vi "Flatten.vi"(6 "Indent":i32, 7 "Linked List in":refnum<class "Linked List.lvclass">, 8 "error in (no error)":errorcluster, 9 "Child IDs":string[](array[string]), 11 "IPersist in":refnum<class "IPersist.lvclass">) -> (0 "error out":errorcluster, 1 "Flattened Linked List":string[](array[string]), 3 "IPersist out":refnum<class "IPersist.lvclass">, 5 "Linked List out":refnum<class "Linked List.lvclass">)   [LabVIEW 2017, in "Linked Lists.lvlib" / "Linked List.lvclass"]
uses:
  <vilib>/gpm_packages/@cs/linked-list/Source/Linked List/Linked List/Linked List.lvclass
  <vilib>/gpm_packages/@cs/persistence/source/IPersist/IPersist.lvclass
  <vilib>/gpm_packages/@cs/linked-list/Source/String Manipulation/String Manipulation.lvlib
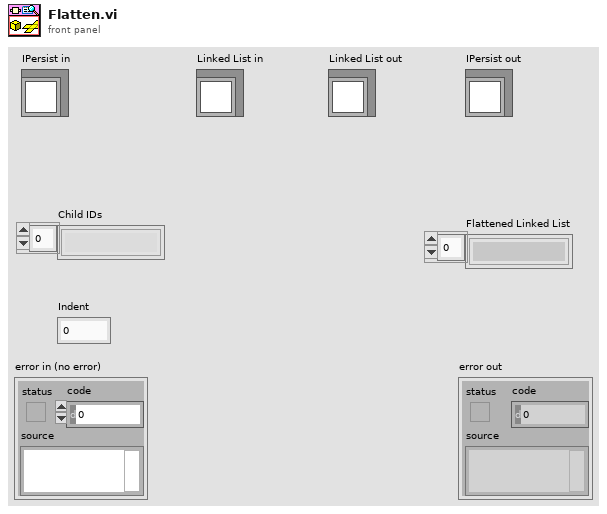
[diagram p1: front panel]
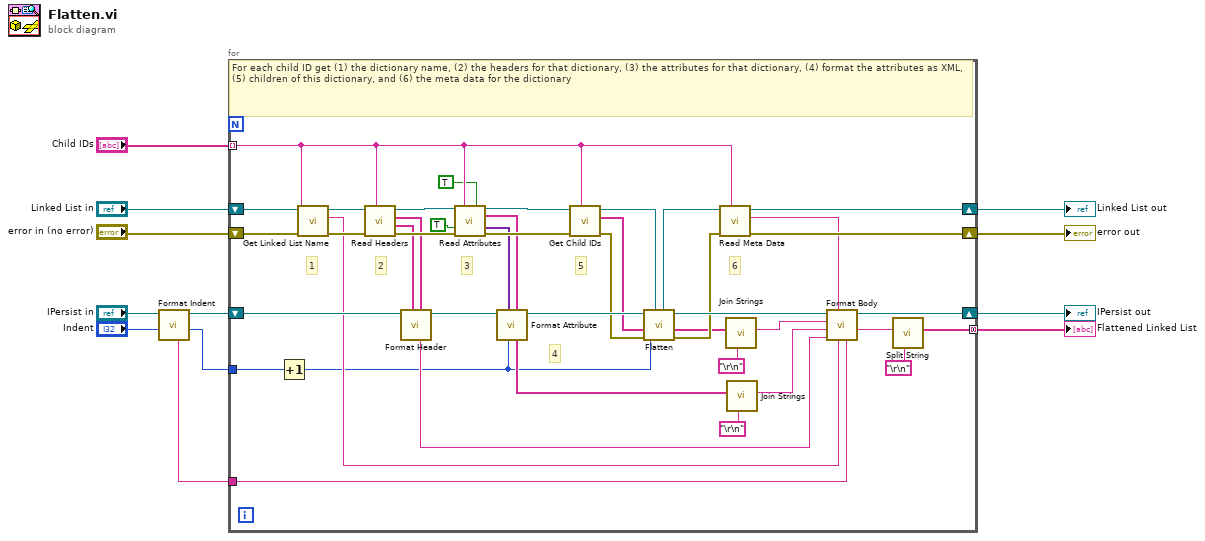
[diagram p0: block diagram]
diagram:
  n1 = call-dynamic "Format Indent.vi"("Indent"="Indent", "IPersist in"="IPersist in") -> ("Indent out"=w11:i32, "IPersist out"=w12:refnum<class "IPersist.lvclass">, "Indent XML"=w10:string)  [unwired: 7 in]
  n2 = for {
    shift-right: [w47] -> w1
    shift-left: "Linked List in" -> [w50]
    shift-right: [w36] -> w3
    shift-left: w12 -> [w45]
    shift-right: [w41] -> w2
    shift-left: "error in (no error)" -> [w49]
    tunnel: w11 -> [w37]
    tunnel: w10 -> [w27]
    tunnel: "Child IDs" -> [w46] mode=indexing
    tunnel: [w25] -> w4 mode=concatenating
    # "4"
    # "6"
    # "5"
    # "3"
    # "2"
    # "1"
    # "For each child ID get (1) the dictionary name, (2) the headers for that dictionary, (3) the attributes for that dictionary, (4) format the attributes as XML, (5) children of this dictionary, and (6) the meta data for the dictionary"
    n3 = Increment(x=w37) -> (x+1=w13:i32)
    n4 = call-dynamic "Get Linked List Name.vi"("error in (no error)"=w49, "Unique ID"=w46, "Linked List in"=w50) -> ("error out"=w53:errorcluster, "Linked List Name"=w28:string, "Linked List out"=w54:refnum<class "Linked List.lvclass">)  [unwired: 5 in, 1 out]
    n5 = call-dynamic "Read Headers.vi"("Linked List ID"=w46, "error in (no error)"=w53, "Linked List in"=w54) -> ("error out"=w51:errorcluster, "Header Values"=w44:string[], "Header Names"=w43:string[], "Linked List out"=w52:refnum<class "Linked List.lvclass">)  [unwired: 4 in, 1 out]
    n6 = call-dynamic "Format Header.vi"("Name"=w43, "Value"=w44, "IPersist in"=w45) -> ("IPersist out"=w40:refnum<class "IPersist.lvclass">, "Header"=w29:string)  [unwired: 7 in]
    n7 = call-dynamic "Read Attributes.vi"("Linked List in"=w52, "Linked List ID"=w46, "Include Private?"=TRUE, "Flatten Pointer?"=TRUE, "error in (no error)"=w51) -> ("Linked List out"=w48:refnum<class "Linked List.lvclass">, "Attribute Names out"=w38:string[], "Attributes"=w39:variant[], "error out"=w42:errorcluster)  [unwired: 4 in, 3 out]
    n8 = call-dynamic "Format Attribute.vi"("Attribute Names"=w38, "Indent"=w13, "Attribute Values"=w39, "IPersist in"=w40) -> ("IPersist out"=w19:refnum<class "IPersist.lvclass">, "Attr Strings"=w31:string[])  [unwired: 6 in]
    n9 = call-dynamic "Get Child IDs.vi"("Linked List ID"=w46, "error in (no error)"=w42, "Linked List in"=w48) -> ("error out"=w17:errorcluster, "Child IDs"=w15:string[], "Linked List out"=w21:refnum<class "Linked List.lvclass">)  [unwired: 6 in]
    n10 = call-dynamic "Flatten.vi"("Indent"=w13, "Linked List in"=w21, "error in (no error)"=w17, "Child IDs"=w15, "IPersist in"=w19) -> ("error out"=w16:errorcluster, "Flattened Linked List"=w14:string[], "IPersist out"=w18:refnum<class "IPersist.lvclass">, "Linked List out"=w20:refnum<class "Linked List.lvclass">)  [unwired: 3 in]
    n11 = call-dynamic "Read Meta Data.vi"("Linked List ID"=w46, "error in (no error)"=w16, "Linked List in"=w20) -> ("error out"=w41:errorcluster, "Meta Data"=w35:string, "Linked List out"=w47:refnum<class "Linked List.lvclass">)  [unwired: 5 in, 1 out]
    n12 = call <vilib>:"Join Strings.vi"("Separator (,)"="\r\n", "Strings In"=w14) -> ("String"=w33:string)  [unwired: 9 in]
    n13 = call <vilib>:"Join Strings.vi"("Separator (,)"="\r\n", "Strings In"=w31) -> ("String"=w30:string)  [unwired: 9 in]
    n14 = call-dynamic "Format Body.vi"("Indent"=w27, "Name"=w28, "Meta Data"=w35, "Header"=w29, "Attributes"=w30, "Body"=w33, "IPersist in"=w18) -> ("String out"=w26:string, "IPersist out"=w36:refnum<class "IPersist.lvclass">)  [unwired: 3 in]
    n15 = call <vilib>:"Split String.vi"("Split Pattern"="\r\n", "Input String"=w26) -> ("Split String"=w25:string[])  [unwired: 9 in]
  }
  "error out" <- w2
  "Linked List out" <- w1
  "IPersist out" <- w3
  "Flattened Linked List" <- w4
